vi "test1-SyncMessage.vi"(8 "error in (no error)":errorcluster, 11 "TestCase in":refnum<class "testcase-CSMMessage.lvclass">) -> (0 "error out":errorcluster, 3 "TestCase out":refnum<class "testcase-CSMMessage.lvclass">)   [LabVIEW 2017, in "testcase-CSMMessage.lvclass"]
uses:
  testcase-CSMMessage.lvclass
  0200cc54-eada-47af-b31a-f532729c858d.vi
  src/user.lib/_NEVSTOP/Communicable State Machine(CSM)/AdvanceAPI/CSM - Make String Arguments Safe.vi
  src/user.lib/_NEVSTOP/Communicable State Machine(CSM)/AdvanceAPI/CSM - Keywords.vi
  <vilib>/addons/_JKI Toolkits/VI Tester/TestCase.llb/TestCase.lvclass
  src/user.lib/_NEVSTOP/Communicable State Machine(CSM)/Communicable State Machine.lvlib
  C:/Program Files (x86)/National Instruments/LabVIEW 2017/vi.lib/addons/_JKI Toolkits/VI Tester/TestCase.llb/TestCase.lvclass
panel:
  out "Loopcount":i32
  out "concatenated string":string
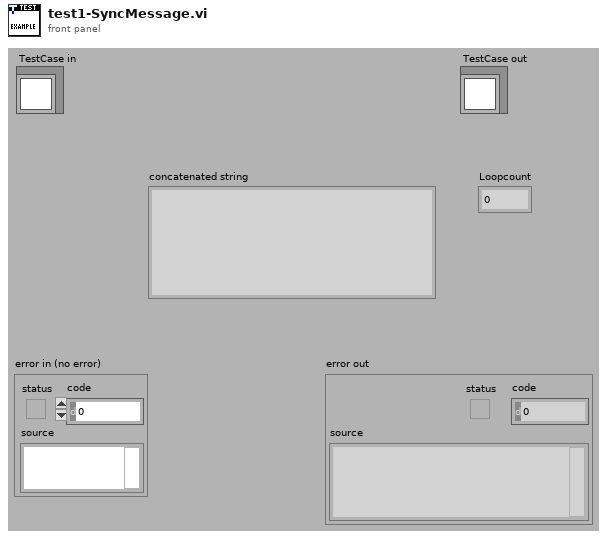
[diagram p1: front panel]
types:
  T1 = cluster{"Arguments":string, "Response":string, "error":errorcluster}
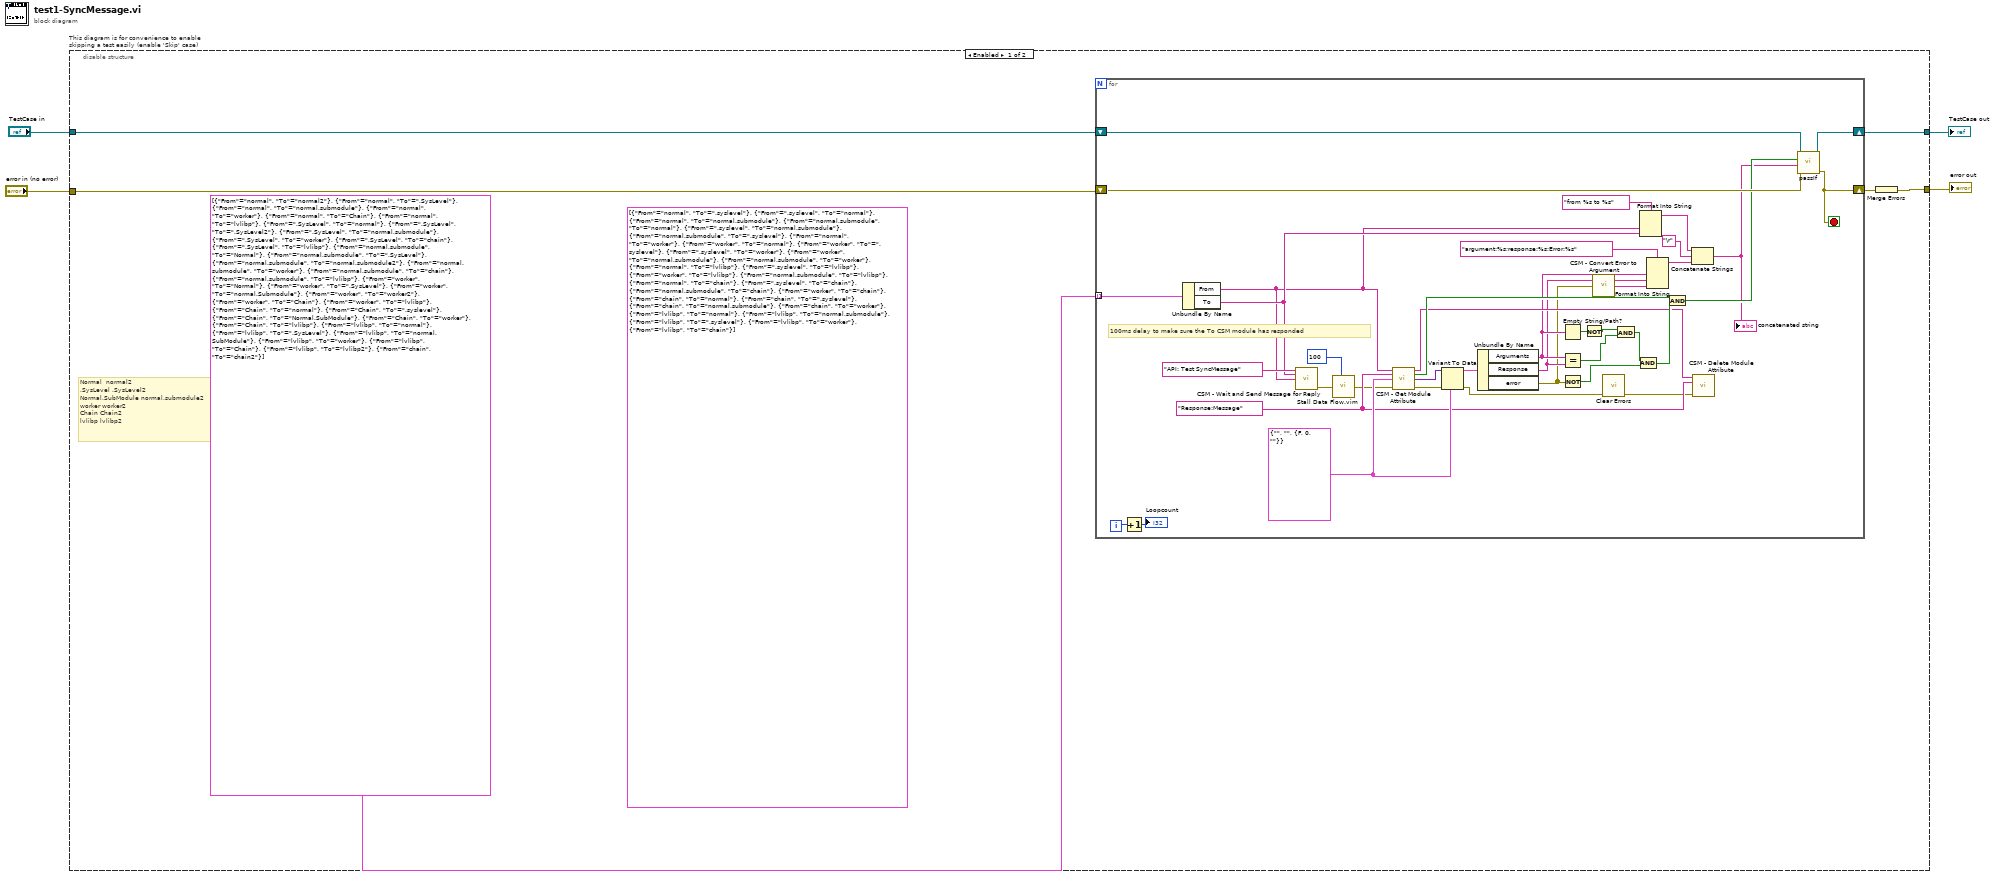
[diagram p0: block diagram]
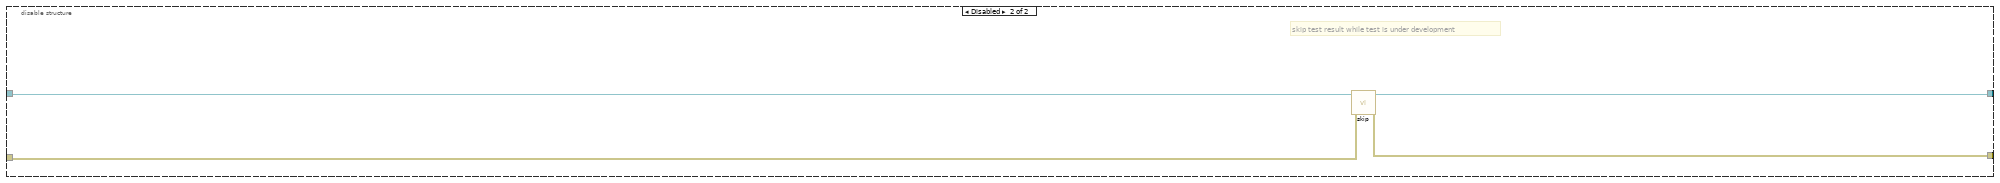
[diagram p2: hidden frame]
diagram:
  n1 = disable-structure "This diagram is for convenience to enable skipping a test easily (enable 'Skip' case)" shown="Enabled" {
    disable-tunnel: "TestCase in" -> [w10 w53]
    disable-tunnel: [w9 w51] -> w1
    disable-tunnel: [w6 w52] -> w3
    disable-tunnel: "error in (no error)" -> [w7 w50]
    frame Enabled {
      (unwired) cluster{"From":string, "To":string}[] [{"From"="normal", "To"=".syslevel"}, {"From"=".syslevel", "To"="normal"}, {"From"="normal", "To"="normal.submodule"}, {"From"="normal.submodule", "To"="normal"}, {"From"=".syslevel", "To"="normal.submodule"}, {"From"="normal.submodule", "To"=".syslevel"}, {"From"="normal", "To"="worker"}, {"From"="worker", "To"="normal"}, {"From"="worker", "To"=".syslevel"}, {"From"=".syslevel", "To"="worker"}, {"From"="worker", "To"="normal.submodule"}, {"From"="normal.submodule", "To"="worker"}, {"From"="normal", "To"="lvlibp"}, {"From"=".syslevel", "To"="lvlibp"}, {"From"="worker", "To"="lvlibp"}, {"From"="normal.submodule", "To"="lvlibp"}, {"From"="normal", "To"="chain"}, {"From"=".syslevel", "To"="chain"}, {"From"="normal.submodule", "To"="chain"}, {"From"="worker", "To"="chain"}, {"From"="chain", "To"="normal"}, {"From"="chain", "To"=".syslevel"}, {"From"="chain", "To"="normal.submodule"}, {"From"="chain", "To"="worker"}, {"From"="lvlibp", "To"="normal"}, {"From"="lvlibp", "To"="normal.submodule"}, {"From"="lvlibp", "To"=".syslevel"}, {"From"="lvlibp", "To"="worker"}, {"From"="lvlibp", "To"="chain"}]
      # "Normal  normal2\n.SysLevel .SysLevel2\nNormal.SubModule normal.submodule2\nworker worker2\nChain Chain2\nlvlibp lvlibp2"
      n2 = for {
        tunnel: cluster{"From":string, "To":string}[] [{"From"="normal", "To"="normal2"}, {"From"="normal", "To"=".SysLevel"}, {"From"="normal", "To"="normal.submodule"}, {"From"="normal", "To"="worker"}, {"From"="normal", "To"="Chain"}, {"From"="normal", "To"="lvlibp"}, {"From"=".SysLevel", "To"="normal"}, {"From"=".SysLevel", "To"=".SysLevel2"}, {"From"=".SysLevel", "To"="normal.submodule"}, {"From"=".SysLevel", "To"="worker"}, {"From"=".SysLevel", "To"="chain"}, {"From"=".SysLevel", "To"="lvlibp"}, {"From"="normal.submodule", "To"="Normal"}, {"From"="normal.submodule", "To"=".SysLevel"}, {"From"="normal.submodule", "To"="normal.submodule2"}, {"From"="normal.submodule", "To"="worker"}, {"From"="normal.submodule", "To"="chain"}, {"From"="normal.submodule", "To"="lvlibp"}, {"From"="worker", "To"="Normal"}, {"From"="worker", "To"=".SysLevel"}, {"From"="worker", "To"="normal.Submodule"}, {"From"="worker", "To"="worker2"}, {"From"="worker", "To"="Chain"}, {"From"="worker", "To"="lvlibp"}, {"From"="Chain", "To"="normal"}, {"From"="Chain", "To"=".syslevel"}, {"From"="Chain", "To"="Normal.SubModule"}, {"From"="Chain", "To"="worker"}, {"From"="Chain", "To"="lvlibp"}, {"From"="lvlibp", "To"="normal"}, {"From"="lvlibp", "To"=".SysLevel"}, {"From"="lvlibp", "To"="normal.SubModule"}, {"From"="lvlibp", "To"="worker"}, {"From"="lvlibp", "To"="Chain"}, {"From"="lvlibp", "To"="lvlibp2"}, {"From"="chain", "To"="chain2"}] -> [w37] mode=indexing
        shift-right: [w48] -> w9
        shift-left: w10 -> [w49]
        shift-right: [w17] -> w8
        shift-left: w7 -> [w47]
        i -> [w12]
        stop <- w17 stop-if-true
        w44 = T1 {"Arguments"="", "Response"="", "error"={"status"=FALSE, "code"=0, "source"=""}}
        w33 = "Response:Message" ("State")
        # "100ms delay to make sure the To CSM module has responded"
        n3 = Increment(x=w12) -> (x+1=→"Loopcount":i32)
        n4 = Unbundle By Name(w37) -> ("From"=w16:string, "To"=w36:string)
        n5 = call "CSM - Wait and Send Message for Reply.vi"("State"="API: Test SyncMessage", "Arguments (\"\")"=w36, "Target Module"=w16) -> ("error out"=w15:errorcluster)  [unwired: 10 in, 2 out]
        n6 = call "Stall Data Flow.vim"("value in"=w15, "milliseconds to wait"=u32 100) -> ("value out"=w14:errorcluster)  [unwired: 1 out]
        n7 = call "CSM - Get Module Attribute.vi"("CSM Name"=w16, "Attribute"=w33, "Default Value (Empty Variant)"=w44, "Error In"=w14) -> ("CSM Name (Dup)"=w34:string, "Found"=w40:bool, "Value"=w43:variant, "error out"=w45:errorcluster)  [unwired: 7 in, 1 out]
        n8 = Variant To Data(error in=w45, type=w44, Variant=w43) -> (data=w42:T1, error out=w19:errorcluster)
        n9 = Unbundle By Name(w42) -> ("Arguments"=w28:string, "Response"=w27:string, "error"=w25:errorcluster)
        n10 = Empty String/Path?(string/path=w28) -> (empty?=w32:bool)
        n11 = Equal?(x=w28, y=w27) -> (x = y?=w30:bool)
        n12 = Not(x=w25) -> (.not. x?=w41:bool)
        n13 = Not(x=w32) -> (.not. x?=w31:bool)
        n14 = call "CSM - Convert Error to Argument.vi"("Error"=w25) -> ("Argument"=w26:string)  [unwired: 4 in]
        n15 = call <vilib>:"Clear Errors.vi"("error in (no error)"=w19) -> ("error out"=w18:errorcluster)  [unwired: 5 in, 1 out]
        n16 = And(x=w31, y=w30) -> (x .and. y?=w29:bool)
        n17 = And(x=w29, y=w41) -> (x .and. y?=w39:bool)
        n18 = Format Into String(format string="from %s to %s", w16, w36) -> (resulting string=w21:string)  [unwired: 2 in, 1 out]
        n19 = Format Into String(format string="argument:%s;response:%s;Error:%s", w28, w27, w26) -> (resulting string=w24:string)  [unwired: 2 in, 1 out]
        n20 = And(x=w40, y=w39) -> (x .and. y?=w38:bool)
        n21 = Concatenate Strings(w21, "\r", w24) -> (w22:string)
        "concatenated string" <- w22
        n22 = call "CSM - Delete Module Attribute.vi"("CSM Name"=w34, "Attribute"=w33, "Error In"=w18) -> ()  [unwired: 9 in, 4 out]
        n23 = call-dynamic "passIf.vi"("error in (no error)"=w47, "message (\"\")"=w22, "pass"=w38, "TestCase in"=w49) -> ("error out"=w17:errorcluster, "TestCase out"=w48:refnum<class "testcase-CSMMessage.lvclass">)  [unwired: 6 in]
      }
      n24 = Merge Errors(w8) -> (w6:errorcluster)
    }
    frame Disabled {
      # "skip test result while test is under development"
      n25 = call <vilib>:"skip.vi"("error in (no error)"=w50, "TestCase in"=w53) -> ("error out"=w52:errorcluster, "TestCase out"=w51:refnum<class "testcase-CSMMessage.lvclass">)  [unwired: 8 in]
    }
  }
  "error out" <- w3
  "TestCase out" <- w1
